vi "Module.Default Tasks.vi"(7 "Sys":T1, 8 "error in":errorcluster, 9 "Data2":variant, 10 "Data1":variant, 11 "Sub":string) -> (0 "error out":errorcluster, 5 "Sys Out":T1)   [LabVIEW 2024, in "EQMF.lvlib" / "Module Utils.lvlib"]
uses:
  Module Utils.lvlib
  Module Sys Info.ctl
  Config/Stored Controls/Class.SaveCtrls.lvclass
  Event Log/Event Notification/Event Notification.lvclass
  Config/App Data/Class.AppData.lvclass
  Subscription/Subscription.lvclass
  Queues/Q.Element.ctl
  Module.SW Version Info.ctl
  Module Config.ctl
  Module.Working Dirs.ctl
  Queues/Queue Utils.lvlib
  Controls/Controls.lvlib
panel:
  # "Name, PN, Version, Note"
  # "Name, PN, Version, Note"
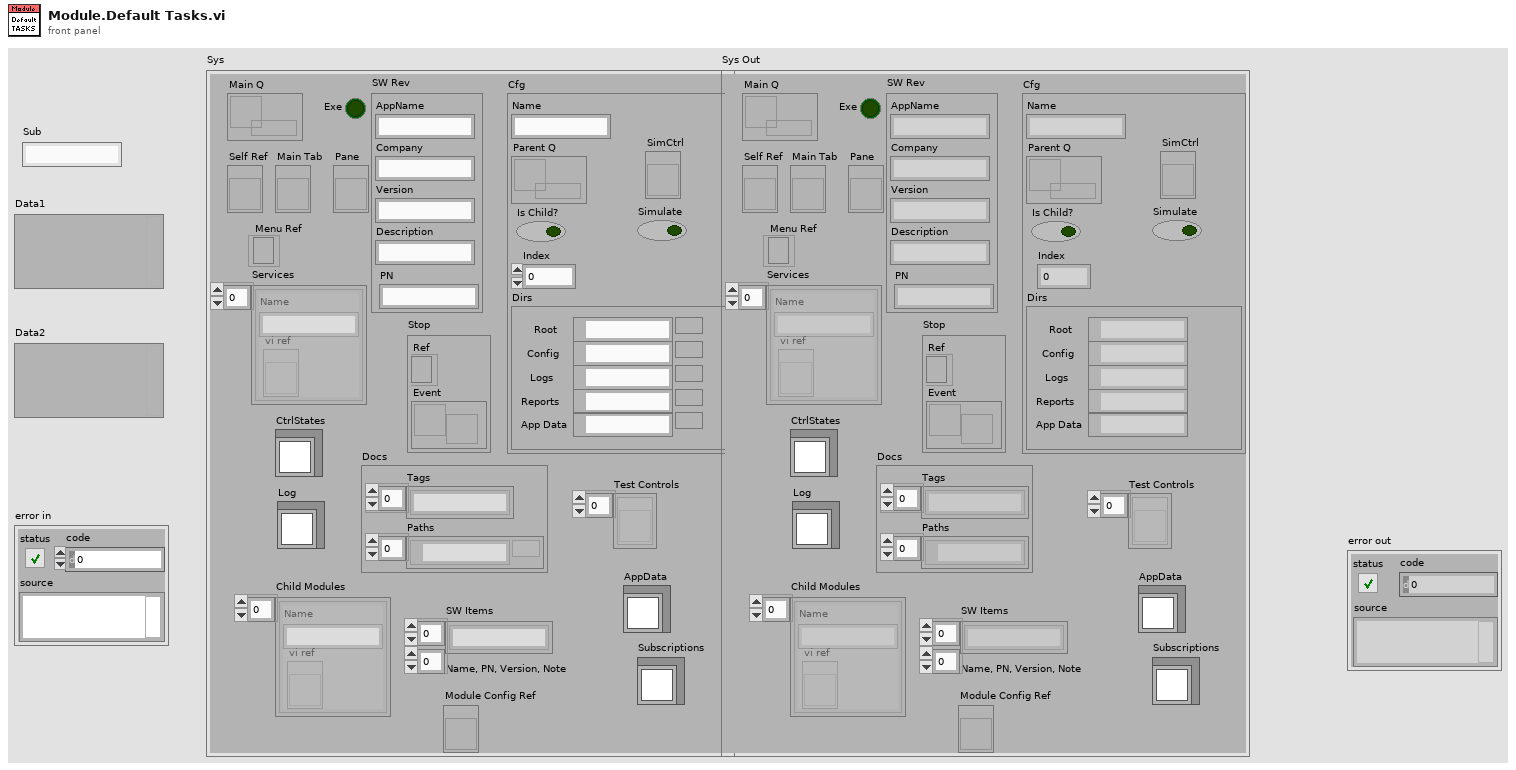
[diagram p1: front panel]
types:
  T1 = typedef "EQMF.lvlib/Module Utils.lvlib/Module Sys Info.ctl" = cluster{"Main Q":refnum<queue>, "Exe":bool, "SW Rev":T2, "Self Ref":refnum<vi>, "Main Tab":refnum<vi>, "Pane":refnum<vi>, "Stop":cluster{"Ref":refnum<event-registration>, "Event":refnum<user-event>}, "Cfg":T3, "Services":cluster{"Name":string, "vi ref":refnum<vi>}[], "Menu Ref":refnum<k9>, "CtrlStates":refnum<class "Class.SaveCtrls.lvclass">, "Docs":cluster{"Tags":string[], "Paths":path[]}, "Log":refnum<class "Event Notification.lvclass">, "Test Controls":refnum<vi>[], "Child Modules":cluster{"Name":string, "vi ref":refnum<vi>}[], "SW Items":string[][], "AppData":refnum<class "Class.AppData.lvclass">, "Subscriptions":refnum<class "Subscription.lvclass">, "Module Config Ref":refnum<vi>}
  T2 = typedef "EQMF.lvlib/Module Utils.lvlib/Module.SW Version Info.ctl" = cluster{"AppName":string, "Company":string, "Version":string, "Description":string, "PN":string}
  T3 = typedef "EQMF.lvlib/Module Utils.lvlib/Module Config.ctl" = cluster{"Name":string, "Parent Q":refnum<queue>, "Is Child?":bool, "Index":i32, "Dirs":T4, "Simulate":bool, "SimCtrl":refnum<vi>}
  T4 = typedef "EQMF.lvlib/Module Utils.lvlib/Module.Working Dirs.ctl" = cluster{"Root":path, "Config":path, "Logs":path, "Reports":path, "App Data":path}
  T5 = enum16{"Top Left", "Bottom Right", "Top Right", "Bottom Left"}
  T6 = typedef "EQMF.lvlib/Queue Utils.lvlib/Q.Element.ctl" = cluster{"Cmd":string, "Sub":string, "Data1":variant, "Data2":variant}
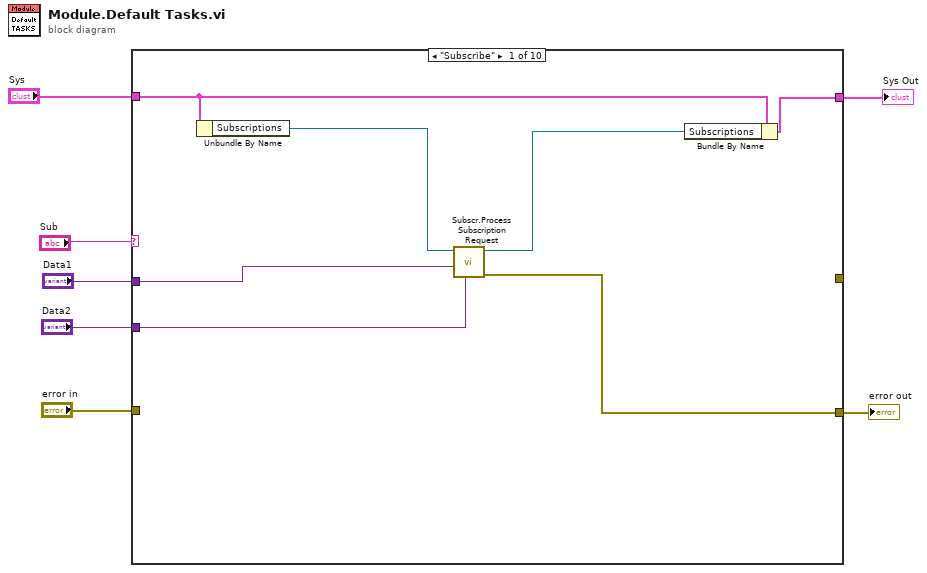
[diagram p0: block diagram]
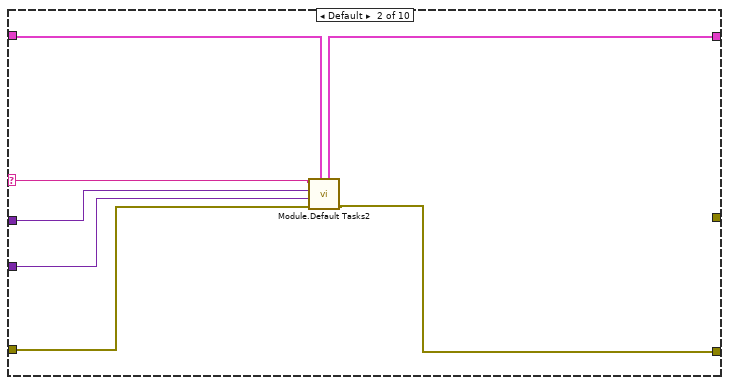
[diagram p2: hidden frame]
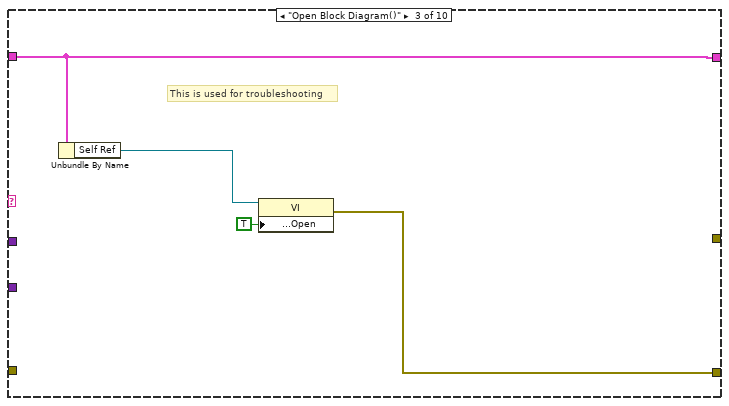
[diagram p3: hidden frame]
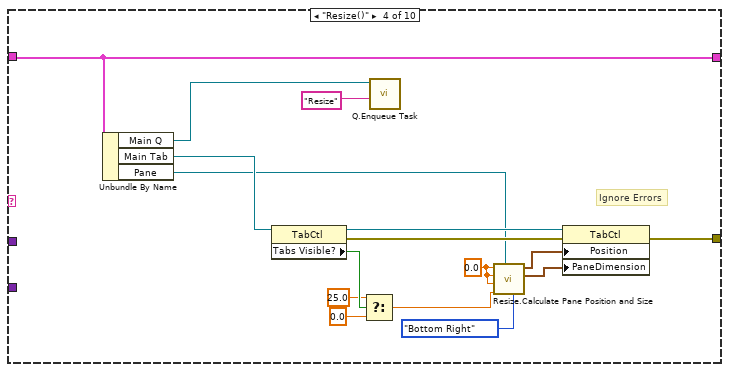
[diagram p4: hidden frame]
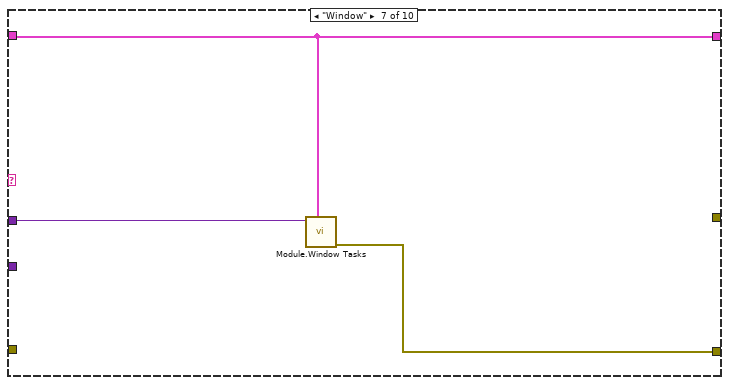
[diagram p7: hidden frame]
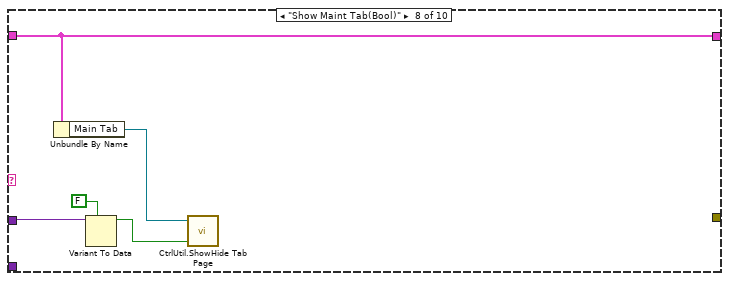
[diagram p8: hidden frame]
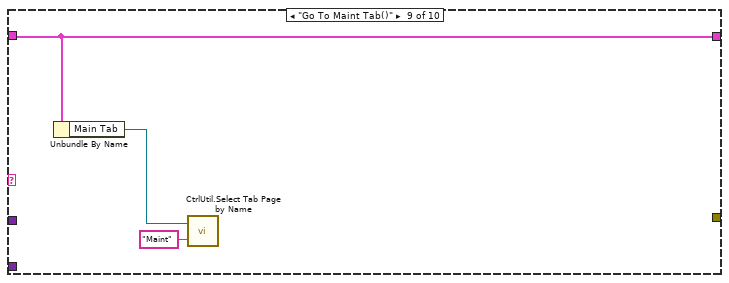
[diagram p9: hidden frame]
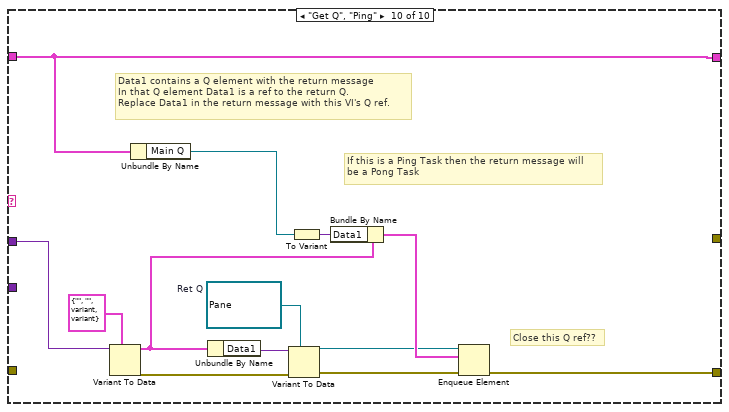
[diagram p10: hidden frame]
diagram:
  n1 = case shown="\"Subscribe\"" "Sub" {
    selector: "Sub" -> [_ w19 _ _ _ _ _ _ _ _]
    tunnel: "Sys" -> [w14 w21 w22 w26 w42 w43 w44 w47 w53 w55]
    tunnel: "Data1" -> [w10 w18 _ _ _ _ w46 w50 _ w66]
    tunnel: "Data2" -> [w9 w17 _ _ _ _ _ _ _ _]
    tunnel: "error in" -> [_ w16 _ _ _ _ _ _ _ _]
    tunnel: [w8 w15 w24 _ _ _ w45 _ _ w67] -> w2
    tunnel: [_ _ _ w29 _ _ _ _ _ _] -> _
    tunnel: [w13 w20 w22 w26 w42 w43 w44 w47 w53 w55] -> w1
    frame "Subscribe" {
      n2 = Unbundle By Name(w14) -> ("Subscriptions"=w12:refnum<class "Subscription.lvclass">)
      n3 = call "Subscr.Process Subscription Request.vi"("Disable(Data2)"=w9, "Request Info (Data1)"=w10, "Subscription in"=w12) -> ("error out"=w8:errorcluster, "Subscription out"=w11:refnum<class "Subscription.lvclass">)  [unwired: 6 in, 1 out]
      n4 = Bundle By Name(cluster=w14, "Subscriptions"=w11) -> (w13:T1)
    }
    frame Default {
      n5 = call "Module.Default Tasks2.vi"("Sys"=w21, "error in"=w16, "Data2"=w17, "Data1"=w18, "Sub"=w19) -> ("error out"=w15:errorcluster, "Sys Out"=w20:T1)  [unwired: 5 in]
    }
    frame "Open Block Diagram()" {
      # "This is used for troubleshooting"
      n6 = Unbundle By Name(w22) -> ("Self Ref"=w23:refnum<vi>)
      n7 = property class="VI"(reference=w23, "Block Diagram Window:Open"=TRUE) -> (error out=w24:errorcluster)  [unwired: 1 in, 1 out]
    }
    frame "Resize()" {
      w32 = 0.0 ("X Origin")
      # "Ignore Errors"
      n8 = Unbundle By Name(w26) -> ("Main Q"=w28:refnum<queue>, "Main Tab"=w41:refnum<vi>, "Pane"=w33:refnum<vi>)
      n9 = property class="TabCtl"(reference=w41) -> (reference out=w40:refnum<vi>, error out=w36:errorcluster, "Tabs Visible?"=w39:bool)  [unwired: 1 in]
      n10 = Select(t=25.0, s=w39, f=0.0) -> (s? t:f=w31:dbl)
      n11 = call "Q.Enqueue Task.vi"("Task Name"="Resize", "Q In"=w28) -> ()  [unwired: 8 in, 2 out]
      n12 = call "Resize.Calculate Pane Position and Size.vi"("Origin for X,Y Max (Top Left)"=T5."Bottom Right", "Pane in"=w33, "Y Max"=w31, "X Max"=w32, "Y Origin"=w32, "X Origin"=w32) -> ("Size"=w34:cluster{u32, u32}, "Position"=w35:cluster{"X Coordinate":i32, "Y Coordinate":i32})  [unwired: 4 in]
      n13 = property class="TabCtl"(reference=w40, error in=w36, "Position"=w35, "PaneDimension"=w34) -> (error out=w29:errorcluster)  [unwired: 1 out]
    }
    frame "Resize" {
      # "If this case is reached then the Task case statement does not have its own \"Resize\" case.\nDo Nothing \n\nIf a VI has something to resize it will have a Task case for Resize and that will be handled there."
    }
    frame "Error Count", "Error Update" {
      # "If this case is reached then the Task case statement does not have its own case.\nDo Nothing"
    }
    frame "Window" {
      n14 = call "Module.Window Tasks.vi"("Sys"=w44, "Data1"=w46) -> ("error out"=w45:errorcluster)  [unwired: 9 in]
    }
    frame "Show Maint Tab(Bool)" {
      n15 = Unbundle By Name(w47) -> ("Main Tab"=w51:refnum<vi>)
      n16 = Variant To Data(type=FALSE, Variant=w50) -> (data=w48:bool)  [unwired: 1 in, 1 out]
      n17 = call "CtrlUtil.ShowHide Tab Page.vi"("Show"=w48, "Tab Control"=w51) -> ()  [unwired: 3 in]
    }
    frame "Go To Maint Tab()" {
      n18 = Unbundle By Name(w53) -> ("Main Tab"=w54:refnum<vi>)
      n19 = call "CtrlUtil.Select Tab Page by Name.vi"("Name"="Maint", "Main Tab"=w54) -> ()  [unwired: 2 in]
    }
    frame "Get Q", "Ping" {
      w56 = refnum<queue> refnum  # Ret Q
      # "Close this Q ref??"
      # "If this is a Ping Task then the return message will\nbe a Pong Task"
      # "Data1 contains a Q element with the return message\nIn that Q element Data1 is a ref to the return Q.\nReplace Data1 in the return message with this VI's Q ref."
      n20 = Variant To Data(type=T6 {"Cmd"="", "Sub"="", "Data1"=variant, "Data2"=variant} ("MainQ.Element"), Variant=w66) -> (data=w57:T6, error out=w64:errorcluster)  [unwired: 1 in]
      n21 = Unbundle By Name(w55) -> ("Main Q"=w61:refnum<queue>)
      n22 = Unbundle By Name(w57) -> ("Data1"=w65:variant)
      n23 = Variant To Data(error in=w64, type=w56, Variant=w65) -> (data=w59:refnum<queue>, error out=w58:errorcluster)
      n24 = To Variant(anything=w61) -> (Variant=w62:variant)
      n25 = Bundle By Name(cluster=w57, "Data1"=w62) -> (w60:T6)
      n26 = Enqueue Element(queue=w59, element=w60, error in (no error)=w58) -> (error out=w67:errorcluster)  [unwired: 1 in, 2 out]
    }
  }
  "error out" <- w2
  "Sys Out" <- w1
